vi "~mmWave prototype.vi"   [LabVIEW 2017]
uses:
  sub-systems/sub-systems.lvclass
  APARMainSubvis/VXM Public API/mmWaveAxis.ctl
  APARMainSubvis/VXM Public API/singleAxisMoveDef.ctl
  VSMx2/VXMx2.lvclass
  MotionComm/MotionComm.lvclass
types:
  T1 = typedef "singleAxisMoveDef.ctl" = cluster{"mmWave Axis":T2, "eng. value":dbl}
  T2 = typedef "mmWaveAxis.ctl" = string
  T3 = typedef "Velmex VXM.lvlib/VXM Axis.ctl" = u16
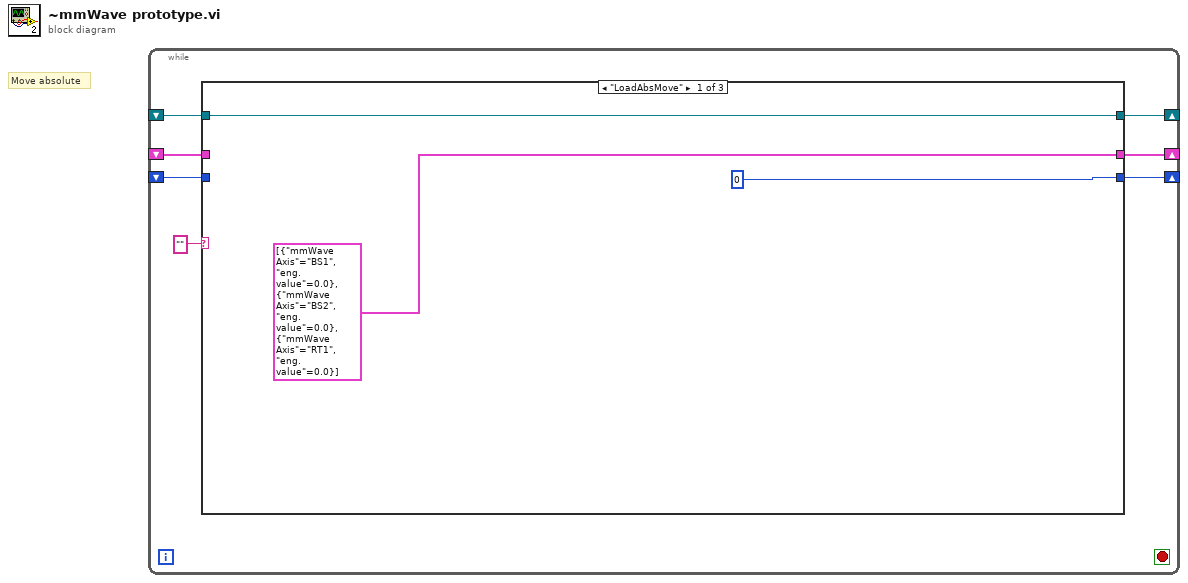
[diagram p0: block diagram]
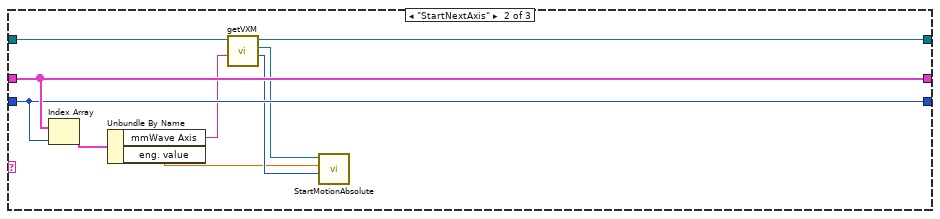
[diagram p2: hidden frame]
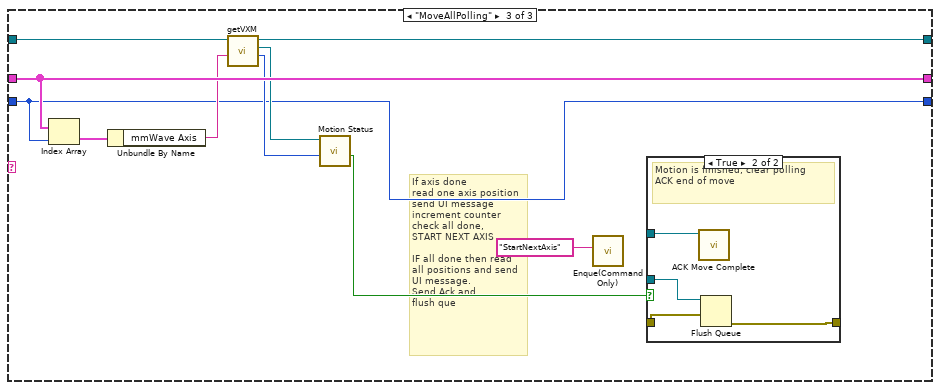
[diagram p3: hidden frame]
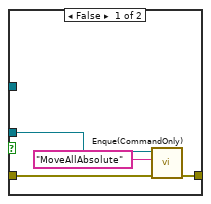
[diagram p4: hidden frame]
diagram:
  # "Move absolute"
  n1 = while {
    shift-right: [w6] -> _
    shift-left: _ -> [w4]
    shift-right: [w5] -> _
    shift-left: _ -> [w3]
    shift-right: [w1] -> _
    shift-left: _ -> [w2]
    stop <- _ stop-if-true
    n2 = case shown="\"LoadAbsMove\"" "" {
      tunnel: [T1[] [{"mmWave Axis"="BS1", "eng. value"=0.0}, {"mmWave Axis"="BS2", "eng. value"=0.0}, {"mmWave Axis"="RT1", "eng. value"=0.0}] ("Position") w19 w29] -> w6
      tunnel: [0 w18 w21] -> w5
      tunnel: w4 -> [_ w19 w29]
      tunnel: w3 -> [_ w18 w21]
      tunnel: w2 -> [w8 w17 w28]
      tunnel: [w8 w16 w27] -> w1
      frame "LoadAbsMove" {
      }
      frame "StartNextAxis" {
        n3 = Index Array(array=w19, index=w18) -> (element=w15:T1)
        n4 = Unbundle By Name(w15) -> ("mmWave Axis"=w14:T2, "eng. value"=w11:dbl)
        n5 = call "getVXM.vi"("mmWave Axis Name"=w14, "sub-systems in"=w17) -> ("Axis (1..4)"=w12:T3, "VXMx2 out"=w13:refnum<class "VXMx2.lvclass">, "sub-systems out"=w16:refnum<class "sub-systems.lvclass">)  [unwired: 5 in, 2 out]
        n6 = call "StartMotionAbsolute.vi"("Axis (1..4)"=w12, "Absolute Position, mm or deg."=w11, "VXMx2 in"=w13) -> ()  [unwired: 7 in, 2 out]
      }
      frame "MoveAllPolling" {
        # "If axis done\nread one axis position\nsend UI message\nincrement counter\ncheck all done,\nSTART NEXT AXIS\n\nIF all done then read\nall positions and send\nUI message.\nSend Ack and \nflush que"
        n7 = Index Array(array=w29, index=w21) -> (element=w26:T1)
        n8 = Unbundle By Name(w26) -> ("mmWave Axis"=w25:T2)
        n9 = call "getVXM.vi"("mmWave Axis Name"=w25, "sub-systems in"=w28) -> ("Axis (1..4)"=w23:T3, "VXMx2 out"=w24:refnum<class "VXMx2.lvclass">, "sub-systems out"=w27:refnum<class "sub-systems.lvclass">)  [unwired: 5 in, 2 out]
        n10 = call "Motion Status.vi"("Axis (1..4)"=w23, "VXMx2 in"=w24) -> ("Motion Stopped"=w22:bool)  [unwired: 6 in, 3 out]
        n11 = call "Enque(CommandOnly).vi"("Message Command"="StartNextAxis" ("Command")) -> ()  [unwired: 9 in, 2 out]
        n12 = case shown="True" w22 {
          tunnel: [w32 w36] -> _
          tunnel: _ -> [w31 w37]
          tunnel: _ -> [w30 w35]
          tunnel: _ -> [_ w34]
          frame False {
            n13 = call "Enque(CommandOnly).vi"("error in"=w31, "Message Command"="MoveAllAbsolute" ("Command"), "Message que"=w30) -> ("error out"=w32:errorcluster)  [unwired: 7 in, 1 out]
          }
          frame True {
            # "Motion is finished, clear polling\nACK end of move"
            n14 = call "ACK Move Complete.vi"("MotionComm in"=w34) -> ()  [unwired: 9 in, 2 out]
            n15 = Flush Queue(queue=w35, error in (no error)=w37) -> (error out=w36:errorcluster)  [unwired: 2 out]
          }
        }
      }
    }
  }
